vi "Measure_Osc_Voltage.vi"(8 "error in":errorcluster) -> (0 "error out":errorcluster, 2 "OscVoltage":dbl)   [LabVIEW 2020]
panel:
  in  "KeyState$":string
  in  "Test String":string
  # "A2B2C1D0F17H0I1M2R31S0T1E"
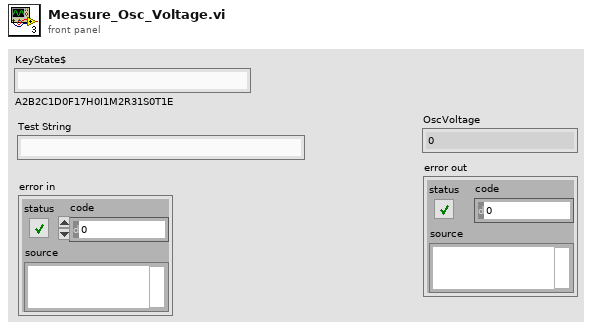
[diagram p1: front panel]
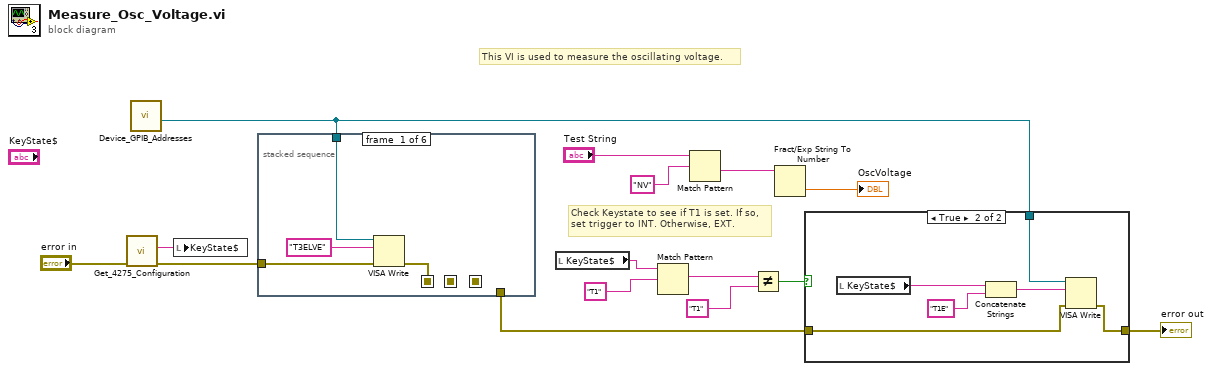
[diagram p0: block diagram]
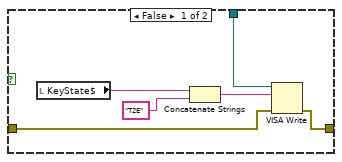
[diagram p2: hidden frame]
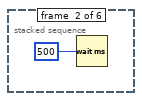
[diagram p3: hidden frame]
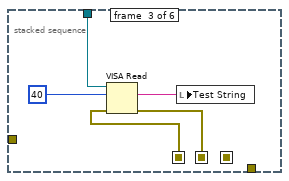
[diagram p4: hidden frame]
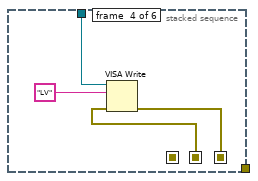
[diagram p5: hidden frame]
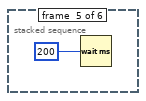
[diagram p6: hidden frame]
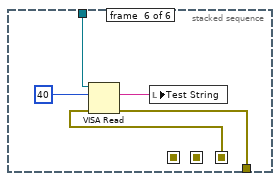
[diagram p7: hidden frame]
diagram:
  # "Check Keystate to see if T1 is set. If so,\nset trigger to INT. Otherwise, EXT."
  # "This VI is used to measure the oscillating voltage."
  n1 = call "Get_4275_Configuration.vi"("error in"="error in") -> ("error out"=w14:errorcluster, "Keystate"=w2:string)  [unwired: 9 in]
  n2 = call "Device_GPIB_Addresses.vi"() -> ("HP 4275A Address"=w1:refnum<visa-resource-name>)  [unwired: 9 in, 2 out]
  n3 = local write "KeyState$"(w2) -> ()
  n4 = stacked-sequence {
    seq-local: [w16 _ _ _ _ _] -> [_ _ w23 _ _ _]
    seq-local: [_ _ w22 _ _ _] -> [_ _ _ w27 _ _]
    seq-local: [_ _ _ w26 _ _] -> [_ _ _ _ _ w32]
    tunnel: w14 -> [w17 _ _ _ _ _]
    tunnel: [_ _ _ _ _ w31] -> w5
    tunnel: w1 -> [w19 _ w25 w29 _ w34]
    frame #0 {
      n5 = VISA Write(VISA resource name=w19, write buffer="T3ELVE" ("data"), error in (no error)=w17) -> (error out=w16:errorcluster)  [unwired: 2 out]
    }
    frame #1 {
      n6 = Wait (ms)(milliseconds to wait=u32 500) -> ()  [unwired: 1 out]
    }
    frame #2 {
      n7 = VISA Read(VISA resource name=w25, byte count=40, error in (no error)=w23) -> (read buffer=w21:string, error out=w22:errorcluster)  [unwired: 2 out]
      n8 = local write "Test String"(w21) -> ()
    }
    frame #3 {
      n9 = VISA Write(VISA resource name=w29, write buffer="LV" ("data"), error in (no error)=w27) -> (error out=w26:errorcluster)  [unwired: 2 out]
    }
    frame #4 {
      n10 = Wait (ms)(milliseconds to wait=u32 200) -> ()  [unwired: 1 out]
    }
    frame #5 {
      n11 = VISA Read(VISA resource name=w34, byte count=40, error in (no error)=w32) -> (read buffer=w35:string, error out=w31:errorcluster)  [unwired: 2 out]
      n12 = local write "Test String"(w35) -> ()
    }
  }
  n13 = local read "KeyState$"() -> (w3:string)
  n14 = Match Pattern(string=w3, regular expression="T1") -> (match substring=w8:string)  [unwired: 1 in, 3 out]
  n15 = Match Pattern(string="Test String", regular expression="NV" ("search string/char (-)")) -> (after substring=w11:string)  [unwired: 1 in, 3 out]
  n16 = Not Equal?(x=w8, y="T1") -> (x != y?=w6:bool)
  n17 = Fract/Exp String To Number(string=w11) -> (number=→"OscVoltage":dbl)  [unwired: 3 in, 1 out]
  n18 = case shown="True" w6 {
    tunnel: w5 -> [w37 w43]
    tunnel: [w36 w42] -> w4
    tunnel: w1 -> [w39 w45]
    frame False {
      n19 = local read "KeyState$"() -> (w40:string)
      n20 = Concatenate Strings(w40, "T2E" ("string")) -> (w38:string)
      n21 = VISA Write(VISA resource name=w39, write buffer=w38, error in (no error)=w37) -> (error out=w36:errorcluster)  [unwired: 2 out]
    }
    frame True {
      n22 = local read "KeyState$"() -> (w46:string)
      n23 = Concatenate Strings(w46, "T1E" ("string")) -> (w44:string)
      n24 = VISA Write(VISA resource name=w45, write buffer=w44, error in (no error)=w43) -> (error out=w42:errorcluster)  [unwired: 2 out]
    }
  }
  "error out" <- w4
